vi "AI Test Temp serial v6.vi"(0 "Command String":string, 5 "Time Out (S)":dbl, 7 "CALIB":dbl) -> (4 "T1":dbl, 6 "T2":dbl, 8 "T3":dbl, 10 "T4":dbl, 13 "error":bool, 14 "output cluster":cluster{dbl, dbl, dbl, dbl, i32, "error #":dbl}, 15 "Unit ID":dbl)   [LabVIEW 2013]
uses:
  <vilib>/Instr/_visa.llb/VISA Configure Serial Port (Instr).vi
panel:
  in  "Loop Time mS":u32
  in  "stop":bool
  in  "Select COM port":refnum<visa-resource-name>
  out "COM port":refnum<visa-resource-name>="COM6"
  out "error #":dbl
  out "End T":dbl
  out "Start T":dbl
  out "read time":dbl
  in  "Array - String":string[](array[string])
  out "end of data (#)":bool
  out "data bytes read":dbl
  out "data string":string
  out "read buffer":string
  out "error out":errorcluster
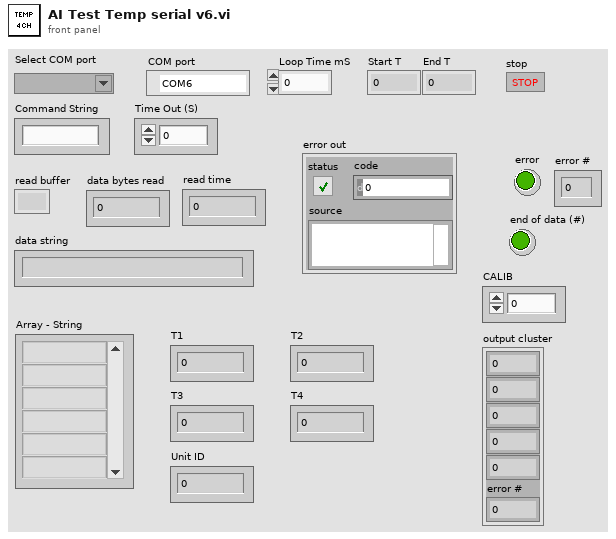
[diagram p1: front panel]
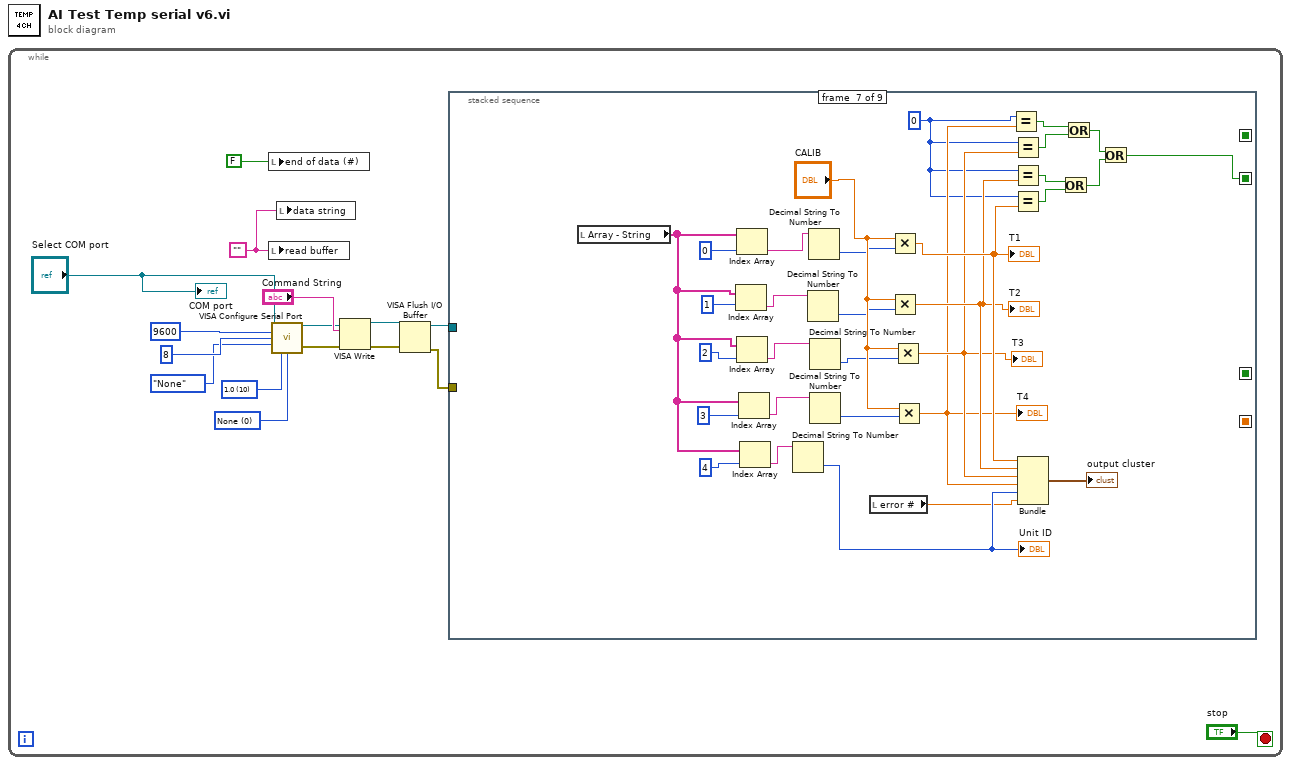
[diagram p0: block diagram]
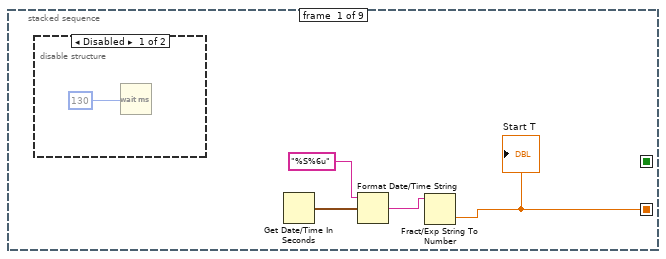
[diagram p2: hidden frame]
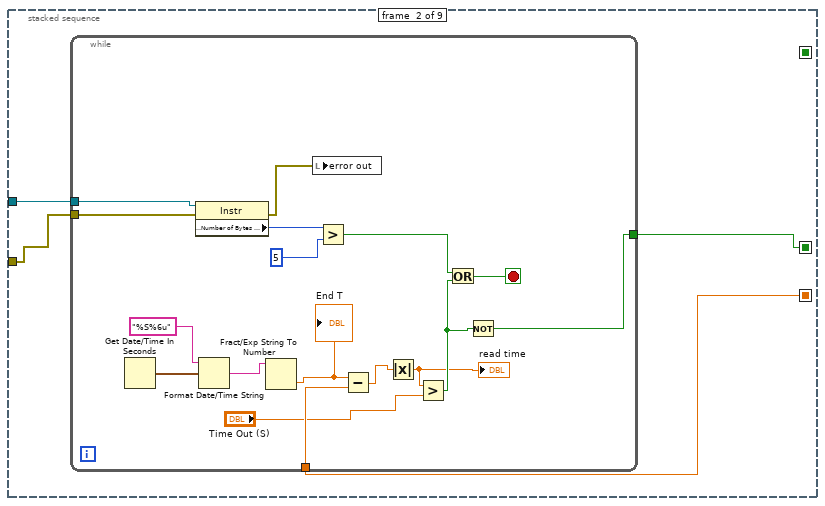
[diagram p4: hidden frame]
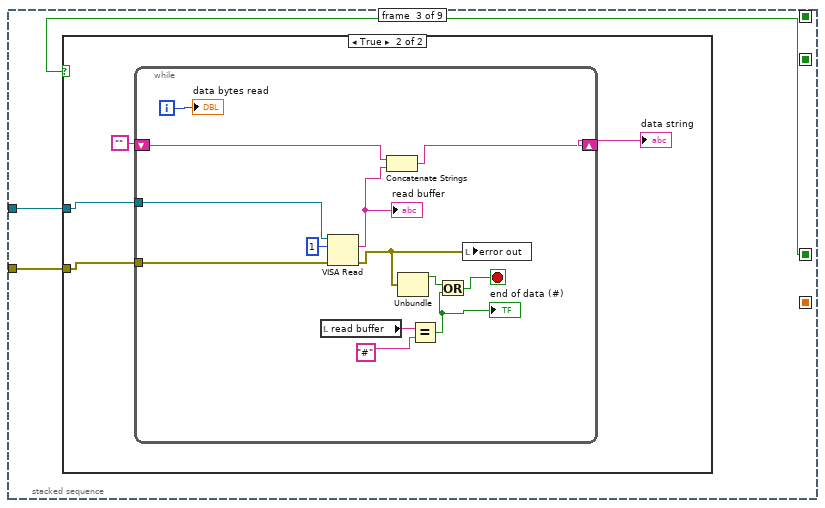
[diagram p5: hidden frame]
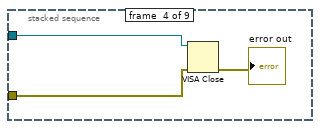
[diagram p7: hidden frame]
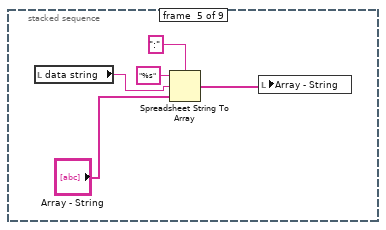
[diagram p8: hidden frame]
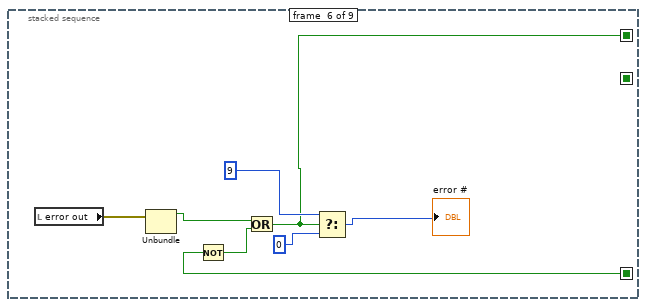
[diagram p9: hidden frame]
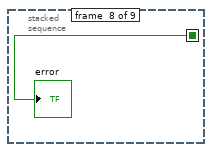
[diagram p10: hidden frame]
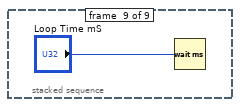
[diagram p11: hidden frame]
diagram:
  n1 = while {
    stop <- "stop" stop-if-true
    w3 = ""
    w12 = u16 0 items=["None", "XON/XOFF", "RTS/CTS", "XON/XOFF & RTS/CTS", "DTR/DSR", "XON/XOFF & DTR/DSR"] ("flow control (0:none)")
    w13 = u16 10 items=["1.0"=10, "1.5"=15, "2.0"=20] ("stop bits (10: 1 bit)")
    n2 = local write "end of data (#)"(FALSE) -> ()
    n3 = local write "read buffer"(w3) -> ()
    n4 = call-poly "VISA Configure Serial Port"("VISA resource name"="Select COM port", "baud rate (9600)"=u32 9600, "data bits (8)"=u16 8, "parity (0:none)"=enum16{"None", "Odd", "Even", "Mark", "Space"}."None", "stop bits (10: 1 bit)"=w13, "flow control (0:none)"=w12) -> ("VISA resource name out"=w5:refnum<visa-resource-name>, "error out"=w4:errorcluster)  [unwired: 8 in]
    n5 = local write "data string"(w3) -> ()
    n6 = VISA Write(VISA resource name=w5, write buffer="Command String", error in (no error)=w4) -> (VISA resource name out=w10:refnum<visa-resource-name>, error out=w9:errorcluster)  [unwired: 1 out]
    n7 = VISA Flush I/O Buffer(VISA resource name=w10, error in (no error)=w9) -> (VISA resource name out=w8:refnum<visa-resource-name>, error out=w7:errorcluster)  [unwired: 1 in]
    n8 = stacked-sequence {
      seq-local: [_ w23 _ _ _ _ _ _ _] -> [_ _ w43 _ _ w76 _ _ _]
      seq-local: [w17 _ _ _ _ _ _ _ _] -> [_ w22 _ _ _ _ _ _ _]
      seq-local: [_ _ _ _ _ w71 _ _ _] -> [_ _ _ _ _ _ _ _ _]
      seq-local: [_ _ _ _ _ _ w79 _ _] -> [_ _ _ _ _ _ _ w110 _]
      tunnel: w8 -> [_ w25 w45 w65 _ _ _ _ _]
      tunnel: w7 -> [_ w24 w44 w64 _ _ _ _ _]
      frame #0 {
        n9 = disable-structure shown="Disabled" {
          frame Disabled {
            n10 = Wait (ms)(milliseconds to wait=130) -> ()  [unwired: 1 out]
          }
          frame Enabled {
          }
        }
        n11 = Get Date/Time In Seconds() -> (seconds since 1Jan1904=w20:timestamp)
        n12 = Format Date/Time String(time format string (%c)="%S%6u", seconds (now)=w20) -> (date/time string=w18:string)  [unwired: 1 in]
        n13 = Fract/Exp String To Number(string=w18) -> (number=w17:dbl)  [unwired: 3 in, 1 out]
        "Start T" <- w17
      }
      frame #1 {
        n14 = while {
          tunnel: w25 -> [w42]
          tunnel: w24 -> [w41]
          tunnel: [w29] -> w23
          tunnel: w22 -> [w33]
          stop <- w31 stop-if-true
          n15 = Get Date/Time In Seconds() -> (seconds since 1Jan1904=w37:timestamp)
          n16 = property class="Instr"(reference=w42, error in=w41) -> (error out=w38:errorcluster, "Serial Settings:Number of Bytes at Serial Port"=w40:u32)  [unwired: 1 out]
          n17 = Format Date/Time String(time format string (%c)="%S%6u", seconds (now)=w37) -> (date/time string=w35:string)  [unwired: 1 in]
          n18 = Fract/Exp String To Number(string=w35) -> (number=w34:dbl)  [unwired: 3 in, 1 out]
          "End T" <- w34
          n19 = local write "error out"(w38) -> ()
          n20 = Greater?(x=w40, y=5) -> (0:w32:bool)
          n21 = Subtract(x=w34, y=w33) -> (x-y=w27:dbl)
          n22 = Absolute Value(x=w27) -> (abs(x)=w26:dbl)
          "read time" <- w26
          n23 = Greater?(x=w26, y="Time Out (S)") -> (0:w30:bool)
          n24 = Or(x=w32, y=w30) -> (x .or. y?=w31:bool)
          n25 = Not(x=w30) -> (.not. x?=w29:bool)
        }
      }
      frame #2 {
        n26 = case shown="True" w43 {
          tunnel: w45 -> [_ w49]
          tunnel: w44 -> [_ w48]
          frame False {
          }
          frame True {
            n27 = while {
              tunnel: w49 -> [w57]
              tunnel: w48 -> [w56]
              shift-right: [w55] -> w47
              shift-left: "" -> [w54]
              i -> [w58]
              stop <- w50 stop-if-true
              n28 = local read "read buffer"() -> (w61:string)
              n29 = VISA Read(VISA resource name=w57, byte count=u32 1, error in (no error)=w56) -> (read buffer=w59:string, error out=w53:errorcluster)  [unwired: 2 out]
              "read buffer" <- w59
              n30 = Concatenate Strings(w54, w59) -> (w55:string)
              n31 = Unbundle(w53) -> ("status"=w52:bool)  [unwired: 2 out]
              n32 = Equal?(x=w61, y="#") -> (x = y?=w51:bool)
              "end of data (#)" <- w51
              n33 = Or(x=w52, y=w51) -> (x .or. y?=w50:bool)
              n34 = local write "error out"(w53) -> ()
              "data bytes read" <- w58
            }
            "data string" <- w47
          }
        }
      }
      frame #3 {
        n35 = VISA Close(VISA resource name=w65, error in (no error)=w64) -> (error out=→"error out":errorcluster)
      }
      frame #4 {
        n36 = local read "data string"() -> (w68:string)
        n37 = Spreadsheet String To Array(delimiter (Tab)=":", format string="%s", spreadsheet string=w68, array type (2D Dbl)="Array - String") -> (array=w66:string[])
        n38 = local write "Array - String"(w66) -> ()
      }
      frame #5 {
        n39 = local read "error out"() -> (w78:errorcluster)
        n40 = Unbundle(w78) -> ("status"=w77:bool)  [unwired: 2 out]
        n41 = Not(x=w76) -> (.not. x?=w75:bool)
        n42 = Or(x=w77, y=w75) -> (x .or. y?=w71:bool)
        n43 = Select(t=9, s=w71, f=0) -> (s? t:f=→"error #":i32)
      }
      frame #6 {
        w86 = 0
        n44 = local read "Array - String"() -> (w101:string[])
        n45 = Index Array(array=w101, index=1) -> (element=w104:string)
        n46 = Index Array(array=w101, index=0) -> (element=w108:string)
        n47 = Index Array(array=w101, index=2) -> (element=w103:string)
        n48 = Index Array(array=w101, index=3) -> (element=w102:string)
        n49 = Index Array(array=w101, index=4) -> (element=w99:string)
        n50 = Decimal String To Number(string=w99) -> (number=w93:i32)  [unwired: 2 in, 1 out]
        "Unit ID" <- w93
        n51 = Decimal String To Number(string=w104) -> (number=w96:i32)  [unwired: 2 in, 1 out]
        n52 = Decimal String To Number(string=w108) -> (number=w97:i32)  [unwired: 2 in, 1 out]
        n53 = Decimal String To Number(string=w103) -> (number=w95:i32)  [unwired: 2 in, 1 out]
        n54 = Decimal String To Number(string=w102) -> (number=w94:i32)  [unwired: 2 in, 1 out]
        n55 = local read "error #"() -> (w92:dbl)
        n56 = Multiply(x="CALIB", y=w97) -> (x*y=w90:dbl)
        "T1" <- w90
        n57 = Multiply(x="CALIB", y=w96) -> (x*y=w89:dbl)
        "T2" <- w89
        n58 = Multiply(x="CALIB", y=w95) -> (x*y=w88:dbl)
        "T3" <- w88
        n59 = Multiply(x="CALIB", y=w94) -> (x*y=w87:dbl)
        "T4" <- w87
        n60 = Equal?(x=w86, y=w87) -> (x = y?=w82:bool)
        n61 = Equal?(x=w86, y=w88) -> (x = y?=w83:bool)
        n62 = Equal?(x=w86, y=w89) -> (x = y?=w85:bool)
        n63 = Equal?(x=w86, y=w90) -> (x = y?=w84:bool)
        n64 = Bundle(w90, w89, w88, w87, w93, "error #"=w92) -> (→"output cluster":cluster{dbl, dbl, dbl, dbl, i32, "error #":dbl})  [unwired: 1 in]
        n65 = Or(x=w85, y=w84) -> (x .or. y?=w80:bool)
        n66 = Or(x=w82, y=w83) -> (x .or. y?=w81:bool)
        n67 = Or(x=w81, y=w80) -> (x .or. y?=w79:bool)
      }
      frame #7 {
        "error" <- w110
      }
      frame #8 {
        n68 = Wait (ms)(milliseconds to wait="Loop Time mS") -> ()  [unwired: 1 out]
      }
    }
    "COM port" <- "Select COM port"
  }
